vi "action.vi"(0 "HGF_FGV_Subset":refnum<class "HGF_FGV_SubSet.lvclass">, 2 "Objects":refnum<class>[](array[class]), 5 "error in (no error)":errorcluster) -> (14 "dup HGF_FGV_Subset":refnum<class "HGF_FGV_SubSet.lvclass">, 16 "dup Objects":refnum<class>[](array[class]), 19 "error out":errorcluster)   [LabVIEW 2012, in "HGF_FGV.lvlib" / "HGF_FGV_SubSet.lvclass"]
doc: "Return copy of addressed objects from object array."
uses:
  HGF_FGV_SubSet.lvclass
  HGF_FGV_SubSet.lvclass/HGF_FGV_SubSet.ctl
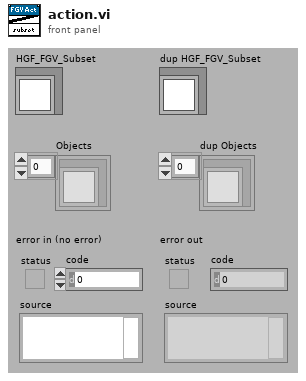
[diagram p1: front panel]
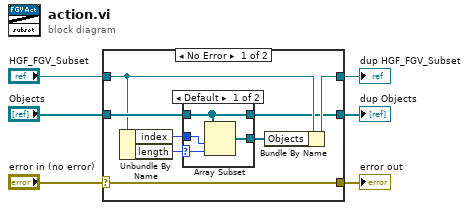
[diagram p0: block diagram]
diagram:
  n1 = case shown="No Error" "error in (no error)" {
    selector: "error in (no error)" -> [w14 w22]
    tunnel: [w14 w22] -> w5
    tunnel: [w9 w21] -> w3
    tunnel: "HGF_FGV_Subset" -> [w10 w21]
    tunnel: [w7 w20] -> w2
    tunnel: "Objects" -> [w12 w20]
    frame No Error {
      n2 = Unbundle By Name(w10) -> ("index"=w13:u32, "length"=w11:i32)
      n3 = case shown="Default" w11 {
        selector: w11 -> [w17 _]
        tunnel: w13 -> [w18 _]
        tunnel: w12 -> [w15 w19]
        tunnel: [w16 w19] -> w8
        tunnel: [w15 w19] -> w7
        frame Default {
          n4 = Array Subset(array=w15, index=w18, length=w17) -> (w16:refnum<class>[])
        }
        frame -1 {
        }
      }
      n5 = Bundle By Name(cluster=w10, "Objects"=w8) -> (w9:refnum<class "HGF_FGV_SubSet.lvclass">)
    }
    frame Error {
    }
  }
  "error out" <- w5
  "dup HGF_FGV_Subset" <- w3
  "dup Objects" <- w2
